vi "SceneObject.vi"(9 "x value 2":dbl format="%0.2f", 10 "x value":dbl format="%0.2f", 11 "SceneObject in":refnum<vi>) -> (3 "SceneObject out":refnum<vi>)   [LabVIEW 2022 SP3]
uses:
  <vilib>/picture/3D Picture Control/NI_3D Picture Control.lvlib
  <vilib>/Analysis/NI_AALPro.lvlib
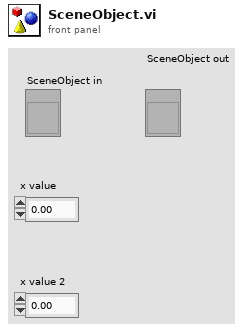
[diagram p1: front panel]
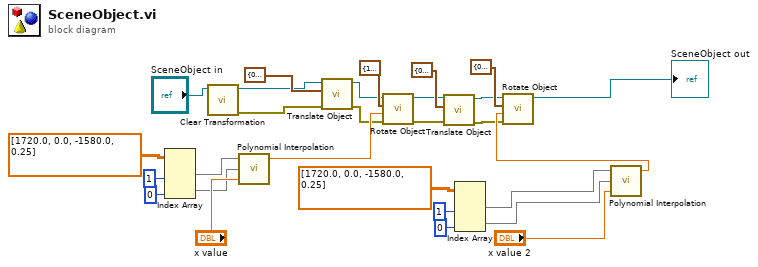
[diagram p0: block diagram]
diagram:
  n1 = Index Array(array=dbl[][] [[1720.0, 0.0], [-1580.0, 0.25]], index (col) #1=1 ("disabled index (col)"), index (col) #2=0 ("index (col)")) -> (element #1=w14:dbl[], element #2=w15:dbl[])  [unwired: 2 in]
  n2 = call <vilib>:"Clear Transformation.vi"("Object Refnum In"="SceneObject in") -> ("error out"=w2:errorcluster, "Object Refnum Out"=w1:refnum<vi>)  [unwired: 9 in]
  n3 = call <vilib>:"Polynomial Interpolation.vi"("x value"="x value", "X"=w15, "Y"=w14) -> ("interpolation value"=w23:dbl)  [unwired: 2 out]
  n4 = call <vilib>:"Translate Object.vi"("error in (no error)"=w2, "Translation"=cluster{"X":sgl, "Y":sgl, "Z":sgl} {"X"=0.0, "Y"=0.0, "Z"=0.0}, "Scene.Object In"=w1) -> ("error out"=w4:errorcluster, "Scene.Object Out"=w3:refnum<vi>)  [unwired: 7 in]
  n5 = call <vilib>:"Rotate Object.vi"("error in (no error)"=w4, "Angle"=w23, "Axis"=cluster{"X":sgl, "Y":sgl, "Z":sgl} {"X"=1.0, "Y"=0.0, "Z"=0.0}, "Scene.Object In"=w3) -> ("error out"=w6:errorcluster, "Scene.Object Out"=w5:refnum<vi>)  [unwired: 6 in]
  n6 = call <vilib>:"Translate Object.vi"("error in (no error)"=w6, "Translation"=cluster{"X":sgl, "Y":sgl, "Z":sgl} {"X"=0.0, "Y"=0.0, "Z"=0.0}, "Scene.Object In"=w5) -> ("error out"=w8:errorcluster, "Scene.Object Out"=w7:refnum<vi>)  [unwired: 7 in]
  n7 = Index Array(array=dbl[][] [[1720.0, 0.0], [-1580.0, 0.25]], index (col) #1=1 ("disabled index (col)"), index (col) #2=0 ("index (col)")) -> (element #1=w20:dbl[], element #2=w21:dbl[])  [unwired: 2 in]
  n8 = call <vilib>:"Polynomial Interpolation.vi"("x value"="x value 2", "X"=w21, "Y"=w20) -> ("interpolation value"=w24:dbl)  [unwired: 2 out]
  n9 = call <vilib>:"Rotate Object.vi"("error in (no error)"=w8, "Angle"=w24, "Axis"=cluster{"X":sgl, "Y":sgl, "Z":sgl} {"X"=0.0, "Y"=0.0, "Z"=1.0}, "Scene.Object In"=w7) -> ("Scene.Object Out"=→"SceneObject out":refnum<vi>)  [unwired: 6 in, 1 out]
